vi "Init.vi"(8 "error in (no error)":errorcluster, 10 "Instrument String":variant, 11 "NI Switch in":refnum<class "NI Switch.lvclass">) -> (0 "error out":errorcluster, 2 "Found?":bool=TRUE, 3 "NI Switch out":refnum<class "NI Switch.lvclass">)   [LabVIEW 2025, in "Switch.lvlib" / "NI Switch.lvclass"]
uses:
  NI Switch.lvclass
  C:/Working copy/tss/Plugin/Engines/Switch/Switch Instrument/Switch Instrument.lvclass
  Switch configuration/Switch configuration.lvclass
  C:/Users/Public/Documents/Sandia National Labs/TSS Plugin/Abstract Engine.lvlibp/Instrument configuration/Instrument configuration.lvclass
  Switch configuration/Switch configuration.lvclass/Switch configuration.ctl
  NI Switch.lvclass/NI Switch.ctl
  Switch configuration/Read Switch Setting.vi
  Users/Public/Documents/Sandia National Labs/TSS Plugin/Abstract Engine.lvlibp/Instrument configuration/Read Instrument Setting.vi
  Users/Public/Documents/Sandia National Labs/TSS Plugin/CEF.lvlibp/serializable configuration/CEF_serializable configuration.lvclass
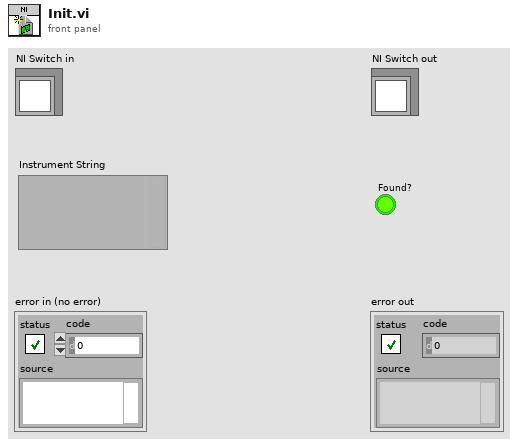
[diagram p1: front panel]
types:
  T1 = typedef "Abstract Engine.lvlibp/Instrument configuration.lvclass/Default Instrument.ctl" = cluster{"Type":string, "Address":string, "SW Alias":string, "Description":string, "Enabled":bool}
  T2 = typedef "Switch.lvlib/Switch configuration.lvclass/Switch Instrument Setting.ctl" = cluster{"topology name":T3}
  T3 = typedef "niSwitch Topologies.ctl" = string
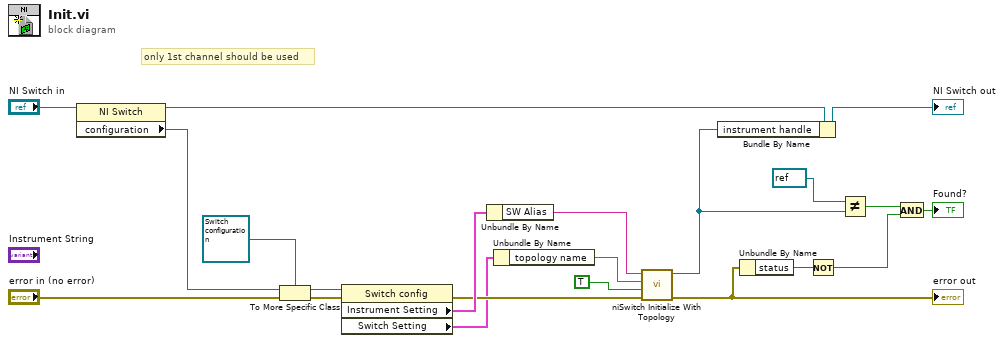
[diagram p0: block diagram]
diagram:
  # "only 1st channel should be used"
  n1 = property class="NI Switch"(reference="NI Switch in") -> (reference out=w19:refnum<class "NI Switch.lvclass">, "configuration"=w17:refnum<class "CEF_serializable configuration.lvclass">)  [unwired: 1 in, 1 out]
  n2 = To More Specific Class(target class=refnum<class "Switch configuration.lvclass"> refnum ("Switch.lvlib:Switch config"), reference=w17, error in="error in (no error)") -> (specific class reference=w18:refnum<class "Switch configuration.lvclass">, error out=w15:errorcluster)
  n3 = property class="Switch config"(reference=w18, error in=w15) -> (error out=w12:errorcluster, "Instrument Setting"=w14:T1, "Switch Setting"=w2:T2)  [unwired: 1 out]
  n4 = Unbundle By Name(w14) -> ("SW Alias"=w11:string)
  n5 = Unbundle By Name(w2) -> ("topology name"=w1:T3)
  n6 = call <instrlib>:"niSwitch Initialize With Topology.vi"("error in (no error)"=w12, "reset device (boolean value)"=TRUE, "topology name"=w1, "resource name"=w11) -> ("error out"=w7:errorcluster, "instrument handle out"=w10:refnum<k15>)  [unwired: 6 in]
  "error out" <- w7
  n7 = Bundle By Name(cluster=w19, "instrument handle"=w10) -> (→"NI Switch out":refnum<class "NI Switch.lvclass">)
  n8 = Unbundle By Name(w7) -> ("status"=w8:bool)
  n9 = Not(x=w8) -> (.not. x?=w5:bool)
  n10 = Not Equal?(x=refnum<k15> refnum ("instrument handle out"), y=w10) -> (x != y?=w6:bool)
  n11 = And(x=w6, y=w5) -> (x .and. y?=→"Found?":bool)
